vi "path coefs.vi"(6 "ypend":dbl, 7 "ypstart":dbl, 8 "yend":dbl=2.0, 9 "ystart":dbl=1.0, 10 "xend":dbl=10.0, 11 "xstart":dbl=1.0) -> (0 "d":dbl, 1 "c":dbl, 2 "b":dbl, 3 "a":dbl)   [LabVIEW 2015]
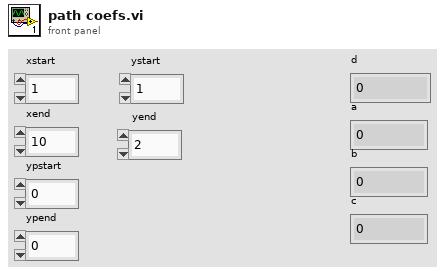
[diagram p1: front panel]
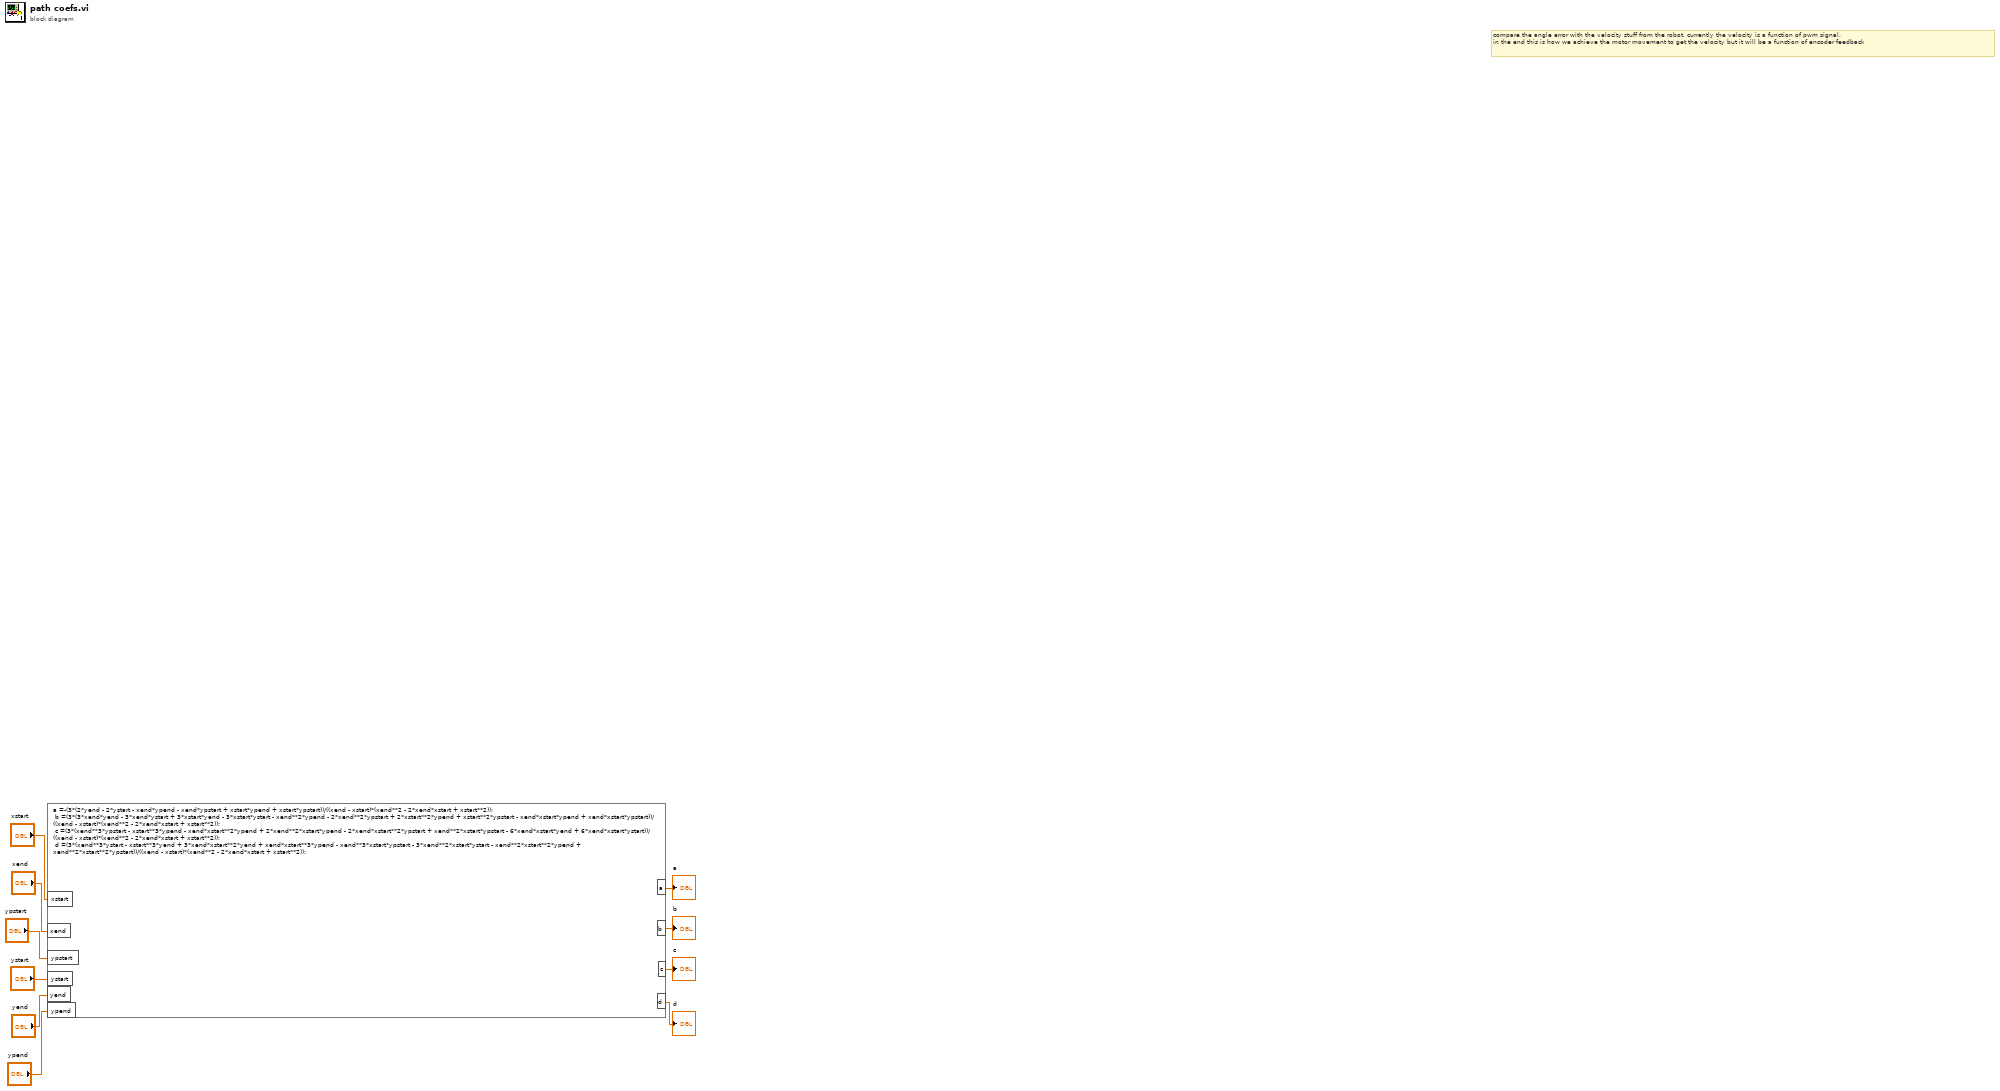
[diagram p0: block diagram]
diagram:
  # "compare the angle error with the velocity stuff from the robot, currently the velocity is a function of pwm signal.\nin the end this is how we achieve the motor movement to get the velocity but it will be a function of encoder feedback"
  n1 = formula code="a =-(3*(2*yend - 2*ystart - xend*ypend - xend*ypstart + xstart*ypend + xstart*ypstart))/((xend - xstart)*(xend**2 - 2*xend*xstart + xstart**2));\n b =(3*(3*xend*yend - 3*xend*ystart + 3*xstart*yend - 3*xstart*ystart - xend**2*ypend - 2*xend**2*ypstart + 2*xstart**2*ypend + xstart**2*ypstart - xend*xstart*ypend + xend*xstart*ypstart))/((xend - xstart)*(xend**2 - 2*xend*xstart + xstart**2));\n c =(3*(xend**3*ypstart - xstart**3*ypend - xend*xstart**2*ypend + 2*xend**2*xstart*ypend - 2*xend*xstart**2*ypstart + xend**2*xstart*ypstart - 6*xend*xstart*yend + 6*xend*xstart*ystart))/((xend - xstart)*(xend**2 - 2*xend*xstart + xstart**2));\n d =(3*(xend**3*ystart - xstart**3*yend + 3*xend*xstart**2*yend + xend*xstart**3*ypend - xend**3*xstart*ypstart - 3*xend**2*xstart*ystart - xend**2*xstart**2*ypend + xend**2*xstart**2*ypstart))/((xend - xstart)*(xend**2 - 2*xend*xstart + xstart**2));"("xstart"="xstart", "xend"="xend", "ypstart"="ypstart", "ystart"="ystart", "yend"="yend", "ypend"="ypend") -> ("a"=→"a":dbl, "b"=→"b":dbl, "c"=→"c":dbl, "d"=→"d":dbl)
